vi "Removes all elements from a queue.vi"(8 "error in (no error)":errorcluster, 11 "Queue name":string) -> (0 "error out":errorcluster)   [LabVIEW 2023, in "Queues.lvlib"]
uses:
  Queues.lvlib
  DUTinfo.ctl
  DUTResult.ctl
  Queue Priority.ctl
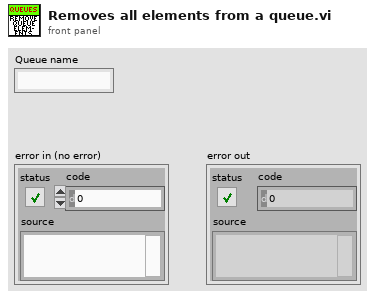
[diagram p1: front panel]
types:
  T1 = typedef "Queues.lvlib/DUTinfo.ctl" = cluster{"Serial Number":string, "Station1":bool, "Station2":bool, "Station3":bool, "Station4":bool, "Acquire Testing":T2, "Queue Priority":T3, "Result_NOKPrint":string[], "SetpointPrint_NOKPrint":string[], "TX_NOKPrint":string[], "RX_NOKPrint":string[], "Daily Number":string}
  T2 = typedef "Queues.lvlib/DUTResult.ctl" = cluster{"IdentNo":string, "Mode":dbl, "CycleTime":dbl, "AttributeSet":string[], "TSNumber":string[], "TSDescription":string[], "TSNominalValueSet":dbl[], "TSLowerToleranceSet":dbl[], "TSUpperToleranceSet":dbl[], "TSUnitSet":string[], "TSValueSet":dbl[], "FailureSet":string[], "FileAttachmentSet":string[]}
  T3 = typedef "Queues.lvlib/Queue Priority.ctl" = enum16{"TOP", "BOTTOM"}
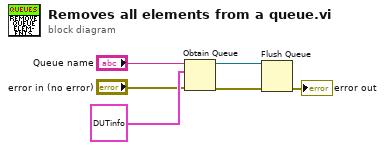
[diagram p0: block diagram]
diagram:
  n1 = Obtain Queue(name (unnamed)="Queue name", element data type=T1 {"Serial Number"="", "Station1"=FALSE, "Station2"=FALSE, "Station3"=FALSE, "Station4"=FALSE, "Acquire Testing"={"IdentNo"="", "Mode"=0.0, "CycleTime"=0.0, "AttributeSet"=[], "TSNumber"=[], "TSDescription"=[], "TSNominalValueSet"=[], "TSLowerToleranceSet"=[], "TSUpperToleranceSet"=[], "TSUnitSet"=[], "TSValueSet"=[], "FailureSet"=[], "FileAttachmentSet"=[]}, "Queue Priority"=enum."TOP", "Result_NOKPrint"=[], "SetpointPrint_NOKPrint"=[], "TX_NOKPrint"=[], "RX_NOKPrint"=[], "Daily Number"=""} ("Element"), error in (no error)="error in (no error)") -> (queue out=w3:refnum<queue>, error out=w2:errorcluster)  [unwired: 2 in, 1 out]
  n2 = Flush Queue(queue=w3, error in (no error)=w2) -> (error out=→"error out":errorcluster)  [unwired: 2 out]
